vi "Follow Path Cascade Helper.vi"(0 "segment":T1, 1 "Encoder Position":dbl, 2 "Encoder Rate":dbl, 3 "Ka":dbl, 4 "Encoder Mean Samples":i32, 6 "Output Range":cluster{"output high":dbl, "output low":dbl}={"output high"=1.0, "output low"=-1.0} {"output low" format="%.2f"; "output high" format="%.2f"}, 7 "i Zone Position":dbl=inf format="%.2f", 8 "i Zone Speed":dbl=inf format="%.2f", 9 "Gains Speed":cluster{"Kp":dbl, "Ki":dbl, "Kd":dbl, "Kf":dbl} {"Kf" format="%.3f"; "Kd" format="%.3f"; "Ki" format="%.3f"; "Kp" format="%.3f"}, 10 "Reinitialize":bool, 11 "Gains Position":cluster{"Kp":dbl, "Ki":dbl, "Kd":dbl, "Kf":dbl} {"Kf" format="%.3f"; "Kd" format="%.3f"; "Ki" format="%.3f"; "Kp" format="%.3f"}) -> (14 "output":dbl, 15 "position output":dbl format="%.2f")   [LabVIEW 2016, in "Drive System.lvlib"]
uses:
  Drive System.lvlib
  Pathfinder/VIs/Segment.ctl
  <vilib>/ptbypt/NI_PtbyPt.lvlib
  Pathfinder/Pathfinder.lvlib
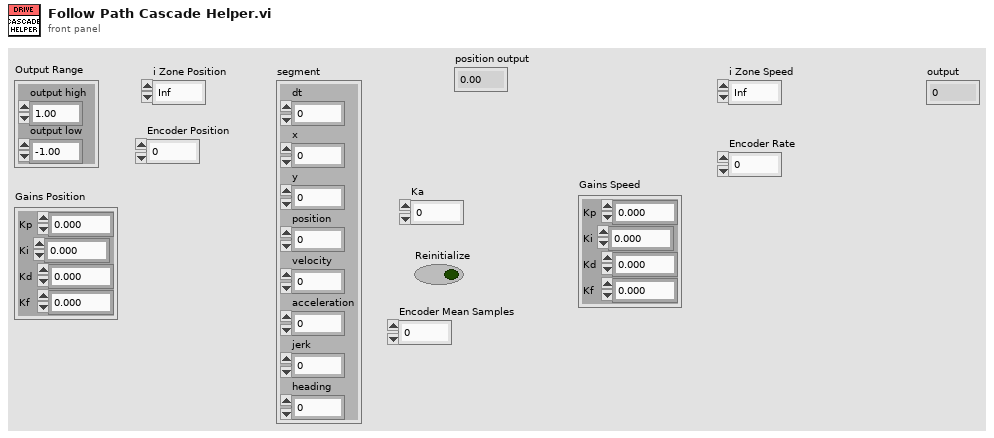
[diagram p1: front panel]
types:
  T1 = typedef "Pathfinder.lvlib/Segment.ctl" = cluster{"dt":dbl, "x":dbl, "y":dbl, "position":dbl, "velocity":dbl, "acceleration":dbl, "jerk":dbl, "heading":dbl}
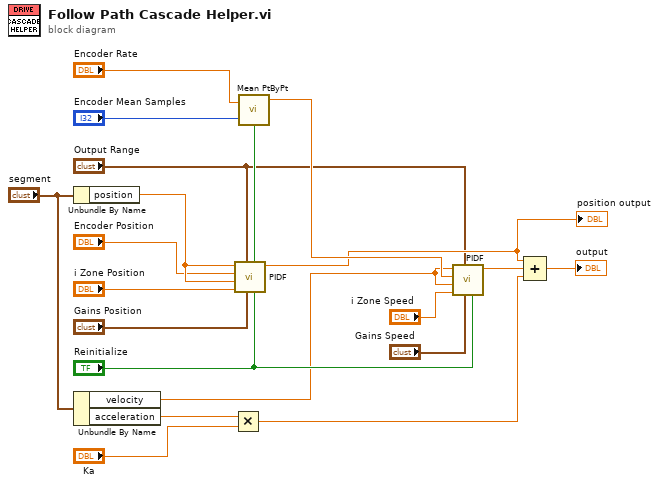
[diagram p0: block diagram]
diagram:
  n1 = Unbundle By Name("segment") -> ("position"=w12:dbl)
  n2 = Unbundle By Name("segment") -> ("velocity"=w5:dbl, "acceleration"=w17:dbl)
  n3 = Multiply(x=w17, y="Ka") -> (x*y=w3:dbl)
  n4 = call "PIDF.vi"("reinitialize? (F)"="Reinitialize", "PIDF gains"="Gains Position", "output range"="Output Range", "i Zone"="i Zone Position", "Feedforward"=w12, "process variable"="Encoder Position", "setpoint"=w12) -> ("output"=w2:dbl)  [unwired: 2 in, 2 out]
  "position output" <- w2
  n5 = call <vilib>:"Mean PtByPt.vi"("x"="Encoder Rate", "sample length"="Encoder Mean Samples", "initialize"="Reinitialize") -> ("mean"=w10:dbl)  [unwired: 1 in, 1 out]
  n6 = call "PIDF.vi"("reinitialize? (F)"="Reinitialize", "PIDF gains"="Gains Speed", "output range"="Output Range", "i Zone"="i Zone Speed", "Feedforward"=w5, "process variable"=w10, "setpoint"=w5) -> ("output"=w19:dbl)  [unwired: 2 in, 2 out]
  n7 = Compound Arithmetic op=ADD(w2, w19, w3) -> (→"output":dbl)
